vi "Autonomous Independent.vi"() -> ()   [LabVIEW 2012]
doc: "This VI is called when autonomous begins, and will automatically be terminated when autonomous ends. You can carry out timed or sensor driven robot movement independently without needing to return to the caller."
uses:
  Robot Global Data.vi
panel:
  in  "intermitend spin-Up":u32=2000
  in  "initSpinUp":u32=10000
  in  "Move Speed":dbl
  in  "Move under time":i32
  in  "Move left/right time":i32
  out "Delay":dbl
  out "Mode":dbl
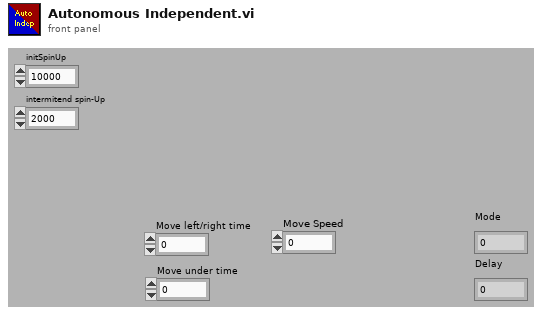
[diagram p1: front panel]
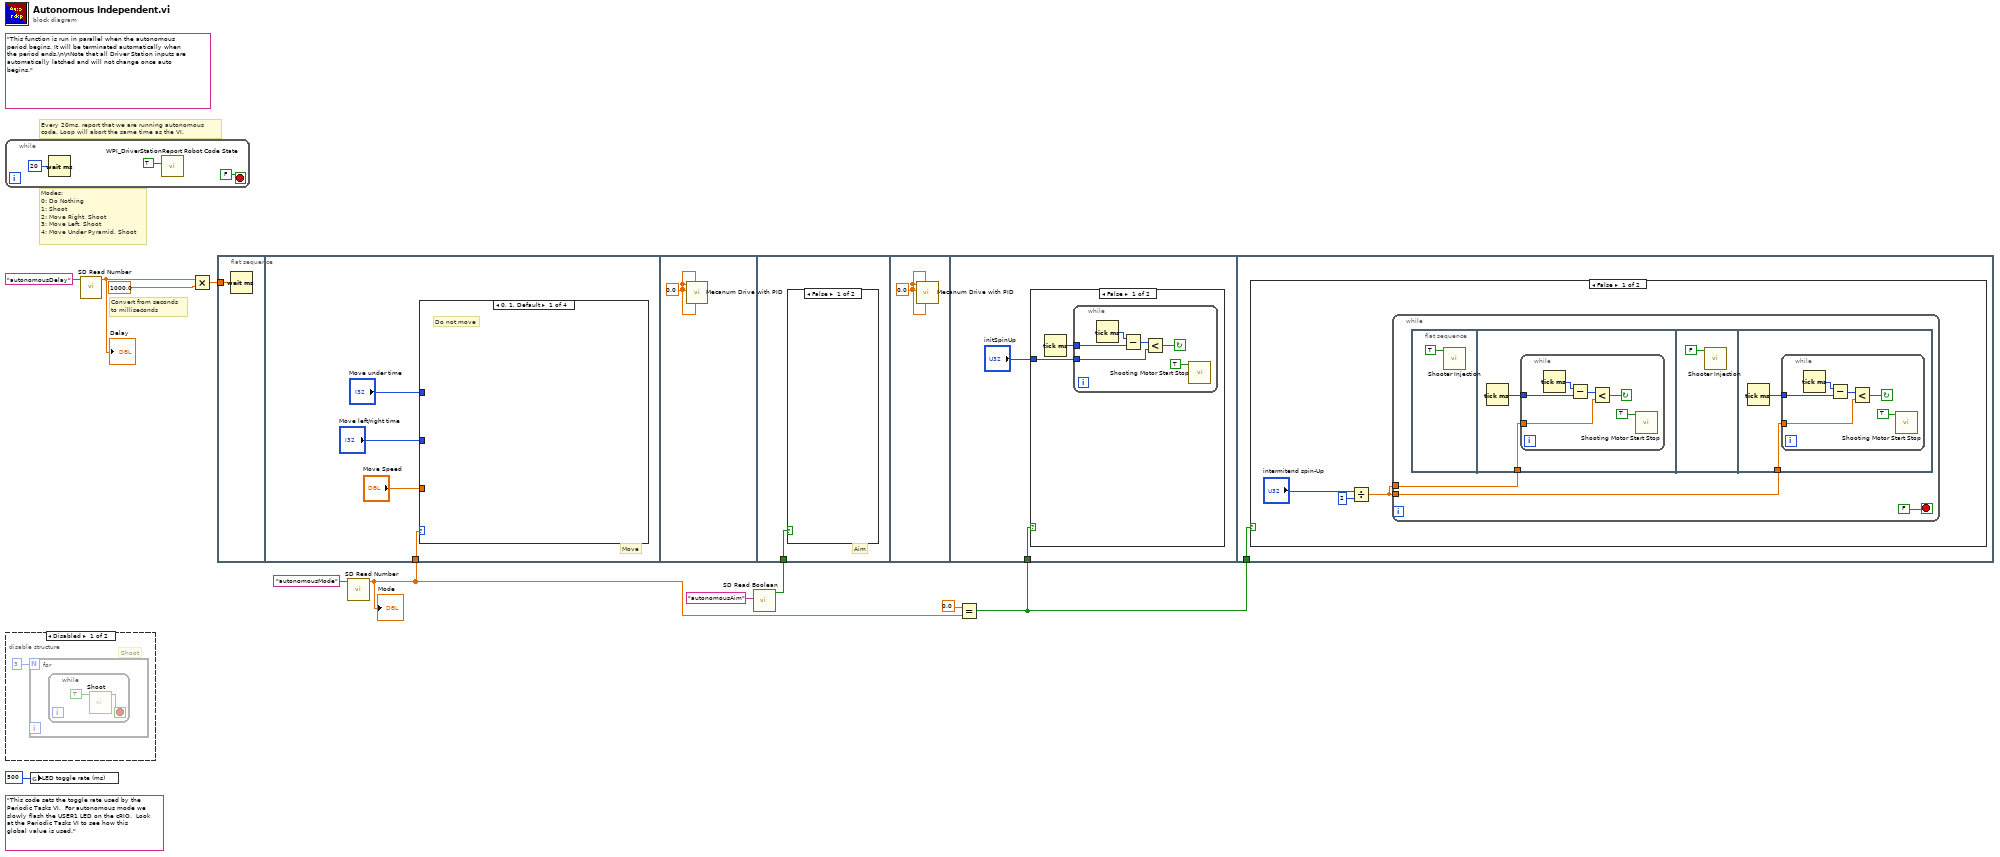
[diagram p0: block diagram]
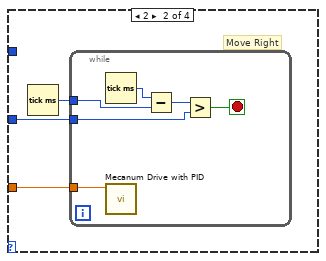
[diagram p3: hidden frame]
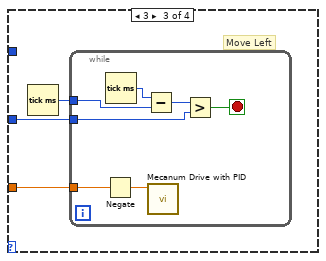
[diagram p4: hidden frame]
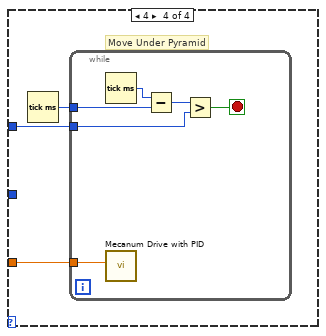
[diagram p5: hidden frame]
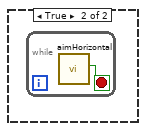
[diagram p6: hidden frame]
diagram:
  (unwired) "This code sets the toggle rate used by the Periodic Tasks VI.  For autonomous mode we slowly flash the USER1 LED on the cRIO.  Look at the Periodic Tasks VI to see how this global value is used."
  (unwired) "This function is run in parallel when the autonomous period begins. It will be terminated automatically when the period ends.\n\nNote that all Driver Station inputs are automatically latched and will not change once auto begins."
  # "Modes:\n0: Do Nothing\n1: Shoot\n2: Move Right, Shoot\n3: Move Left, Shoot\n4: Move Under Pyramid, Shoot"
  # "Convert from seconds\nto milliseconds"
  # "Every 20ms, report that we are running autonomous\ncode. Loop will abort the same time as the VI."
  n1 = while {
    stop <- FALSE stop-if-true
    n2 = Wait (ms)(milliseconds to wait=u32 20) -> ()  [unwired: 1 out]
    n3 = call <vilib>:"WPI_DriverStationReport Robot Code State.vi"("Autonomous"=TRUE) -> ()  [unwired: 10 in, 1 out]
  }
  n4 = disable-structure shown="Disabled" {
    frame Disabled {
      # "Shoot"
      n5 = for {
        N: 3 -> [_]
        n6 = while {
          stop <- w16 stop-if-true
          n7 = call "Shoot.vi"("startShooting"=TRUE) -> ("Done"=w16:bool)  [unwired: 10 in]
        }
      }
    }
    frame Enabled {
    }
  }
  n8 = global write "Robot Global Data.vi" "LED toggle rate (ms)"(u32 500 ("LED ms toggle rate")) -> ()
  n9 = call <vilib>:"SD Read Number.vi"("Name"="autonomousDelay") -> ("Numeric"=w7:dbl)  [unwired: 8 in, 2 out]
  "Delay" <- w7
  n10 = Multiply(x=w7, y=1000.0) -> (x*y=w9:dbl)
  n11 = flat-sequence {
    tunnel: w9 -> [w18]
    tunnel: w3 -> [w22]
    tunnel: w4 -> [w52]
    tunnel: w1 -> [w55]
    tunnel: w1 -> [w65]
    frame #0 {
      n12 = Wait (ms)(milliseconds to wait=w18) -> ()  [unwired: 1 out]
    }
    frame #1 {
      # "Move"
      n13 = case shown="0, 1, Default" w22 {
        tunnel: "Move left/right time" -> [_ w24 w33 _]
        tunnel: "Move under time" -> [_ _ _ w43]
        tunnel: "Move Speed" -> [_ w23 w32 w42]
        frame 0, 1, Default {
          # "Do not move"
        }
        frame 2 {
          # "Move Right"
          n14 = Tick Count (ms)() -> (millisecond timer value=w25:u32)
          n15 = while {
            tunnel: w25 -> [w30]
            tunnel: w24 -> [w27]
            tunnel: w23 -> [w26]
            stop <- w29 stop-if-true
            n16 = Tick Count (ms)() -> (millisecond timer value=w31:u32)
            n17 = call "Mecanum Drive with PID.vi"("X"=w26) -> ()  [unwired: 11 in]
            n18 = Subtract(x=w31, y=w30) -> (x-y=w28:u32)
            n19 = Greater?(x=w28, y=w27) -> (0:w29:bool)
          }
        }
        frame 3 {
          # "Move Left"
          n20 = Tick Count (ms)() -> (millisecond timer value=w34:u32)
          n21 = while {
            tunnel: w34 -> [w40]
            tunnel: w33 -> [w37]
            tunnel: w32 -> [w35]
            stop <- w39 stop-if-true
            n22 = Negate(x=w35) -> (-x=w36:dbl)
            n23 = Tick Count (ms)() -> (millisecond timer value=w41:u32)
            n24 = Subtract(x=w41, y=w40) -> (x-y=w38:u32)
            n25 = call "Mecanum Drive with PID.vi"("X"=w36) -> ()  [unwired: 11 in]
            n26 = Greater?(x=w38, y=w37) -> (0:w39:bool)
          }
        }
        frame 4 {
          # "Move Under Pyramid"
          n27 = Tick Count (ms)() -> (millisecond timer value=w44:u32)
          n28 = while {
            tunnel: w44 -> [w49]
            tunnel: w43 -> [w46]
            tunnel: w42 -> [w45]
            stop <- w48 stop-if-true
            n29 = Tick Count (ms)() -> (millisecond timer value=w50:u32)
            n30 = call "Mecanum Drive with PID.vi"("Y"=w45) -> ()  [unwired: 11 in]
            n31 = Subtract(x=w50, y=w49) -> (x-y=w47:u32)
            n32 = Greater?(x=w47, y=w46) -> (0:w48:bool)
          }
        }
      }
    }
    frame #2 {
      w51 = 0.0 ("Gyro Angle")
      n33 = call "Mecanum Drive with PID.vi"("Rotation"=w51, "MaxSpeed"=w51, "Y"=w51, "X"=w51) -> ()  [unwired: 8 in]
    }
    frame #3 {
      # "Aim"
      n34 = case shown="False" w52 {
        frame False {
        }
        frame True {
          n35 = while {
            stop <- w53 stop-if-true
            n36 = call "aimHorizontal.vi"() -> ("Done"=w53:bool)  [unwired: 11 in]
          }
        }
      }
    }
    frame #4 {
      w54 = 0.0 ("Gyro Angle")
      n37 = call "Mecanum Drive with PID.vi"("Rotation"=w54, "MaxSpeed"=w54, "Y"=w54, "X"=w54) -> ()  [unwired: 8 in]
    }
    frame #5 {
      n38 = case shown="False" w55 {
        tunnel: "initSpinUp" -> [w57 _]
        frame False {
          n39 = Tick Count (ms)() -> (millisecond timer value=w58:u32)
          n40 = while {
            tunnel: w58 -> [w63]
            tunnel: w57 -> [w60]
            stop <- w62 continue-if-true
            n41 = Tick Count (ms)() -> (millisecond timer value=w64:u32)
            n42 = Subtract(x=w64, y=w63) -> (x-y=w61:u32)
            n43 = Less?(x=w61, y=w60) -> (x < y?=w62:bool)
            n44 = call "Shooting Motor Start Stop.vi"("Start"=TRUE) -> ()  [unwired: 10 in, 1 out]
          }
        }
        frame True {
        }
      }
    }
    frame #6 {
      n45 = case shown="False" w65 {
        frame False {
          n46 = Divide(x="intermitend spin-Up", y=u32 2) -> (x/y=w66:dbl)
          n47 = while {
            tunnel: w66 -> [w71]
            tunnel: w66 -> [w70]
            stop <- FALSE stop-if-true
            n48 = flat-sequence {
              tunnel: w71 -> [w73]
              tunnel: w70 -> [w82]
              frame #0 {
                n49 = call "Shooter Injection.vi"("Inject"=TRUE) -> ()  [unwired: 11 in]
              }
              frame #1 {
                n50 = Tick Count (ms)() -> (millisecond timer value=w74:u32)
                n51 = while {
                  tunnel: w74 -> [w79]
                  tunnel: w73 -> [w77]
                  stop <- w76 continue-if-true
                  n52 = Tick Count (ms)() -> (millisecond timer value=w80:u32)
                  n53 = Subtract(x=w80, y=w79) -> (x-y=w78:u32)
                  n54 = Less?(x=w78, y=w77) -> (x < y?=w76:bool)
                  n55 = call "Shooting Motor Start Stop.vi"("Start"=TRUE) -> ()  [unwired: 10 in, 1 out]
                }
              }
              frame #2 {
                n56 = call "Shooter Injection.vi"("Inject"=FALSE) -> ()  [unwired: 11 in]
              }
              frame #3 {
                n57 = Tick Count (ms)() -> (millisecond timer value=w83:u32)
                n58 = while {
                  tunnel: w83 -> [w88]
                  tunnel: w82 -> [w85]
                  stop <- w86 continue-if-true
                  n59 = Tick Count (ms)() -> (millisecond timer value=w89:u32)
                  n60 = Subtract(x=w89, y=w88) -> (x-y=w87:u32)
                  n61 = Less?(x=w87, y=w85) -> (x < y?=w86:bool)
                  n62 = call "Shooting Motor Start Stop.vi"("Start"=TRUE) -> ()  [unwired: 10 in, 1 out]
                }
              }
            }
          }
        }
        frame True {
          # "mode=0\nDo nothing"
        }
      }
    }
  }
  n63 = call <vilib>:"SD Read Number.vi"("Name"="autonomousMode") -> ("Numeric"=w3:dbl)  [unwired: 8 in, 2 out]
  "Mode" <- w3
  n64 = call <vilib>:"SD Read Boolean.vi"("Table Prefix"="autonomousAim" ("Name")) -> ("Boolean"=w4:bool)  [unwired: 8 in, 2 out]
  n65 = Equal?(x=0.0, y=w3) -> (x = y?=w1:bool)
